vi "Callback - Grow.vi"(11 "Growable Widget In":refnum<class "LQObject.lvclass">) -> ()   [LabVIEW 2013, in "Growable Widget.lvclass"]
uses:
  Growable Widget.lvclass
  src/LabVIEW/LQ Core/LQObject/LQObject.lvclass
  Growable Widget.lvclass/Growable Widget.ctl
  Widget Builders/Abstract Widget Builder/Abstract Widget Builder.lvclass
  Widget Builders/Tab Widget Builder/Tab Widget Builder.lvclass
  Widget Builders/Tool Box Builder/Tool Box Builder.lvclass
  Widget Builders/Splitter Builder/Splitter Builder.lvclass
  src/LabVIEW/LQ Core/Qt/Orientation.ctl
  Widget Builders/Splitter Builder/Splitter Builder.lvclass/Splitter Builder.ctl
  Widget Builders/MDI Area Builder/MDI Area Builder.lvclass
  src/LabVIEW/Qt Widgets/QWidget/QWidget.lvclass
  src/LabVIEW/Qt Widgets/QComboBox/QComboBox.lvclass
  src/LabVIEW/Qt Widgets/QLineEdit/QLineEdit.lvclass
  src/LabVIEW/LQ Core/Qt/Qt.lvlib
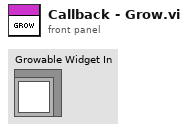
[diagram p1: front panel]
types:
  T1 = typedef "Qt.lvlib/Orientation.ctl" = i32
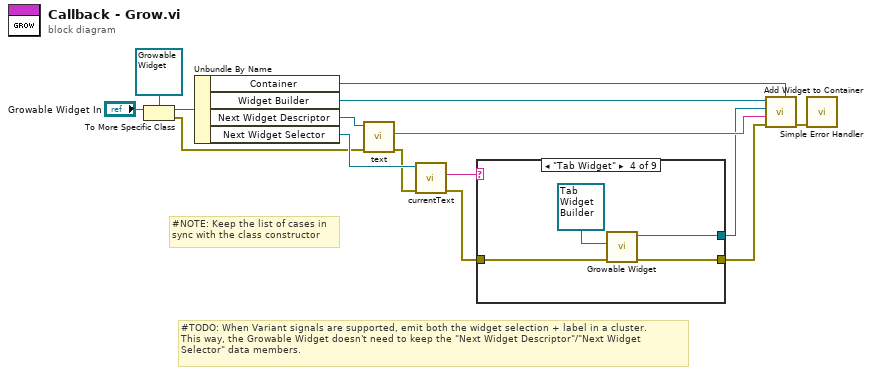
[diagram p0: block diagram]
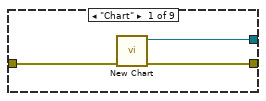
[diagram p2: hidden frame]
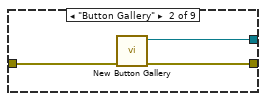
[diagram p3: hidden frame]
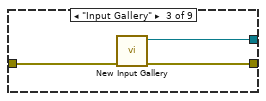
[diagram p4: hidden frame]
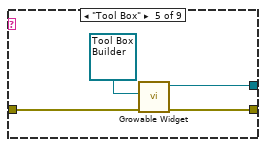
[diagram p5: hidden frame]
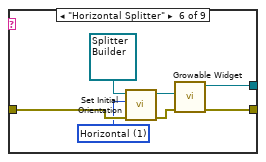
[diagram p6: hidden frame]
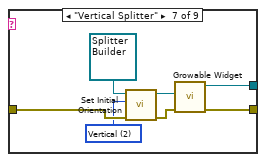
[diagram p7: hidden frame]
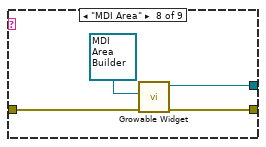
[diagram p8: hidden frame]
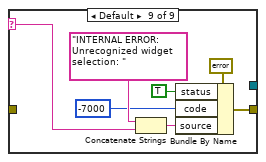
[diagram p9: hidden frame]
diagram:
  # "#NOTE: Keep the list of cases in\nsync with the class constructor"
  # "#TODO: When Variant signals are supported, emit both the widget selection + label in a cluster.\nThis way, the Growable Widget doesn't need to keep the \"Next Widget Descriptor\"/\"Next Widget\nSelector\" data members."
  n1 = To More Specific Class(target class=refnum<class "Growable Widget.lvclass"> refnum ("Growable Widget.lvclass"), reference="Growable Widget In") -> (specific class reference=w13:refnum<class "Growable Widget.lvclass">, error out=w2:errorcluster)  [unwired: 1 in]
  n2 = Unbundle By Name(w13) -> ("Container"=w11:refnum<class "QWidget.lvclass">, "Widget Builder"=w12:refnum<class "Abstract Widget Builder.lvclass">, "Next Widget Descriptor"=w10:refnum<class "QLineEdit.lvclass">, "Next Widget Selector"=w4:refnum<class "QComboBox.lvclass">)
  n3 = call "text.vi"("Error In"=w2, "QLineEdit In"=w10) -> ("Error Out"=w1:errorcluster, "Value"=w9:string)  [unwired: 7 in, 1 out]
  n4 = call "currentText.vi"("Error In"=w1, "QComboBox In"=w4) -> ("Error Out"=w3:errorcluster, "Value"=w8:string)  [unwired: 7 in, 1 out]
  n5 = case shown="\"Tab Widget\"" w8 {
    selector: w8 -> [_ _ _ _ _ _ _ _ w56]
    tunnel: [w16 w19 w23 w27 w29 w39 w46 w48 _] -> w7
    tunnel: w3 -> [w18 w21 w24 w26 w31 w37 w44 w50 _]
    tunnel: [w17 w20 w22 w25 w30 w38 w45 w47 w51] -> w6
    frame "Chart" {
      n6 = call "New Chart.vi"("Error In"=w18) -> ("Error Out"=w17:errorcluster, "New LQChart"=w16:refnum<class "LQChart.lvclass">)  [unwired: 9 in]
    }
    frame "Button Gallery" {
      n7 = call "New Button Gallery.vi"("Error In"=w21) -> ("Error Out"=w20:errorcluster, "New Button Gallery"=w19:refnum<class "QWidget.lvclass">)  [unwired: 9 in]
    }
    frame "Input Gallery" {
      n8 = call "New Input Gallery.vi"("Error In"=w24) -> ("Error Out"=w22:errorcluster, "New Input Gallery"=w23:refnum<class "QWidget.lvclass">)  [unwired: 9 in]
    }
    frame "Tab Widget" {
      n9 = call "Growable Widget.vi"("Error In"=w26, "Widget Builder"=refnum<class "Tab Widget Builder.lvclass"> refnum ("Tab Widget Builder.lvclass")) -> ("Error Out"=w25:errorcluster, "New Growable Widget"=w27:refnum<class "Growable Widget.lvclass">)  [unwired: 8 in]
    }
    frame "Tool Box" {
      n10 = call "Growable Widget.vi"("Error In"=w31, "Widget Builder"=refnum<class "Tool Box Builder.lvclass"> refnum ("Tool Box Builder.lvclass")) -> ("Error Out"=w30:errorcluster, "New Growable Widget"=w29:refnum<class "Growable Widget.lvclass">)  [unwired: 8 in]
    }
    frame "Horizontal Splitter" {
      w33 = T1 1 items=["Horizontal"=1, "Vertical"=2] ("Orientation")
      n11 = call "Set Initial Orientation.vi"("Error In"=w37, "Initial Orientation"=w33, "Splitter Builder in"=refnum<class "Splitter Builder.lvclass"> refnum ("Splitter Builder.lvclass")) -> ("Error Out"=w36:errorcluster, "Splitter Builder out"=w34:refnum<class "Splitter Builder.lvclass">)  [unwired: 7 in]
      n12 = call "Growable Widget.vi"("Error In"=w36, "Widget Builder"=w34) -> ("Error Out"=w38:errorcluster, "New Growable Widget"=w39:refnum<class "Growable Widget.lvclass">)  [unwired: 8 in]
    }
    frame "Vertical Splitter" {
      w40 = T1 2 items=["Horizontal"=1, "Vertical"=2] ("Orientation")
      n13 = call "Set Initial Orientation.vi"("Error In"=w44, "Initial Orientation"=w40, "Splitter Builder in"=refnum<class "Splitter Builder.lvclass"> refnum ("Splitter Builder.lvclass")) -> ("Error Out"=w43:errorcluster, "Splitter Builder out"=w41:refnum<class "Splitter Builder.lvclass">)  [unwired: 7 in]
      n14 = call "Growable Widget.vi"("Error In"=w43, "Widget Builder"=w41) -> ("Error Out"=w45:errorcluster, "New Growable Widget"=w46:refnum<class "Growable Widget.lvclass">)  [unwired: 8 in]
    }
    frame "MDI Area" {
      n15 = call "Growable Widget.vi"("Error In"=w50, "Widget Builder"=refnum<class "MDI Area Builder.lvclass"> refnum ("MDI Area Builder.lvclass")) -> ("Error Out"=w47:errorcluster, "New Growable Widget"=w48:refnum<class "Growable Widget.lvclass">)  [unwired: 8 in]
    }
    frame Default {
      n16 = Concatenate Strings("INTERNAL ERROR: Unrecognized widget selection: ", w56) -> (w53:string)
      n17 = Bundle By Name(cluster=errorcluster {"status"=FALSE, "code"=0, "source"=""} ("Error Out"), "status"=TRUE, "code"=-7000, "source"=w53) -> (w51:errorcluster)
    }
  }
  n18 = call-dynamic "Add Widget to Container.vi"("Container"=w11, "Error In"=w6, "Label"=w9, "Widget"=w7, "Abstract Widget Builder in"=w12) -> ("Error Out"=w5:errorcluster)  [unwired: 5 in, 1 out]
  n19 = call <vilib>:"Simple Error Handler.vi"("error in (no error)"=w5) -> ()  [unwired: 4 in, 5 out]
